vi "Apply ROIs.vi"(5 "Function":T1=enum."Write-from dataset", 7 "Mode (Redraw All)":enum16{"Redraw All", "Draw Last"}(ring), 8 "error in (no error)":errorcluster, 9 "ROIs Info []":T2[](array[typedef]) {"Zoom" min=1.0 max=10.0 step=0.10000000149011612}) -> (0 "error out":errorcluster, 1 "Number of ROI":i32, 2 "Cycle time (us)":dbl, 3 "No ROI":bool)   [LabVIEW 2017]
uses:
  Typedefs/ROI spec.ctl
  Typedefs/ROI ID Enum.ctl
  Typedefs/ROI management FG states.ctl
  Typedefs/ROI management Input cluster.ctl
  Global Variables/General Globals.vi
  <resource>/objmgr/IMAQImage.rc
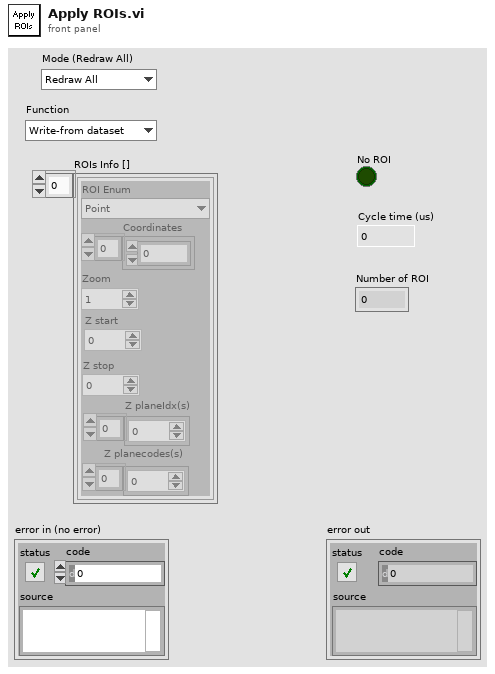
[diagram p1: front panel]
types:
  T1 = typedef "ROI management FG states.ctl" = enum16{"Read", "Write", "Write-from dataset", "Clear Last", "Clear All", "Update ROIs time", "Reload last ROI set", "Offset all ROI", "Offset visible ROI"}
  T2 = typedef "ROI spec.ctl" = cluster{"Coordinates":i32[], "Zoom":dbl, "ROI Enum":T3, "Z planeIdx(s)":i32[], "Z planecodes(s)":u8[], "Z start":dbl, "Z stop":dbl}
  T3 = typedef "ROI ID Enum.ctl" = enum16{"Point", "MiniScan", "Comp. MiniScan", "Rectangle", "Comp. volume", "Arb. plane point", "None"}
  T4 = typedef "ROI parameters data type.ctl" = cluster{"ROI index":dbl, "ROI ID":dbl, "ROI Time (ns)":dbl, "Pixels in ROI":dbl, "X start":dbl, "Y start":dbl, "Z start":dbl, "X stop":dbl, "Y stop":dbl, "Z stop":dbl, "Angle (deg)":dbl, "Composite ID":dbl, "Number of lines":dbl, "Frame Size":dbl, "Zoom":dbl, "Laser Power (%)":dbl, "ROI group ID":dbl, "Z Plane Idx":i32[], "Z Plane codes":i32[]}
  T5 = typedef "ROI management Input cluster.ctl" = cluster{"ROI Type":T3, "XY Coordinates":i32[], "Motor Z Planes":dbl[], "Dwell time per POI or per pixel (us)":dbl, "Frame size":i32, "Zoom":dbl, "Z Plane Idx(s)":i32[], "Z Plane codes":u8[], "Z start":dbl, "Z stop":dbl}
  T6 = typedef "IMAQ Image.ctl" = refnum<image>
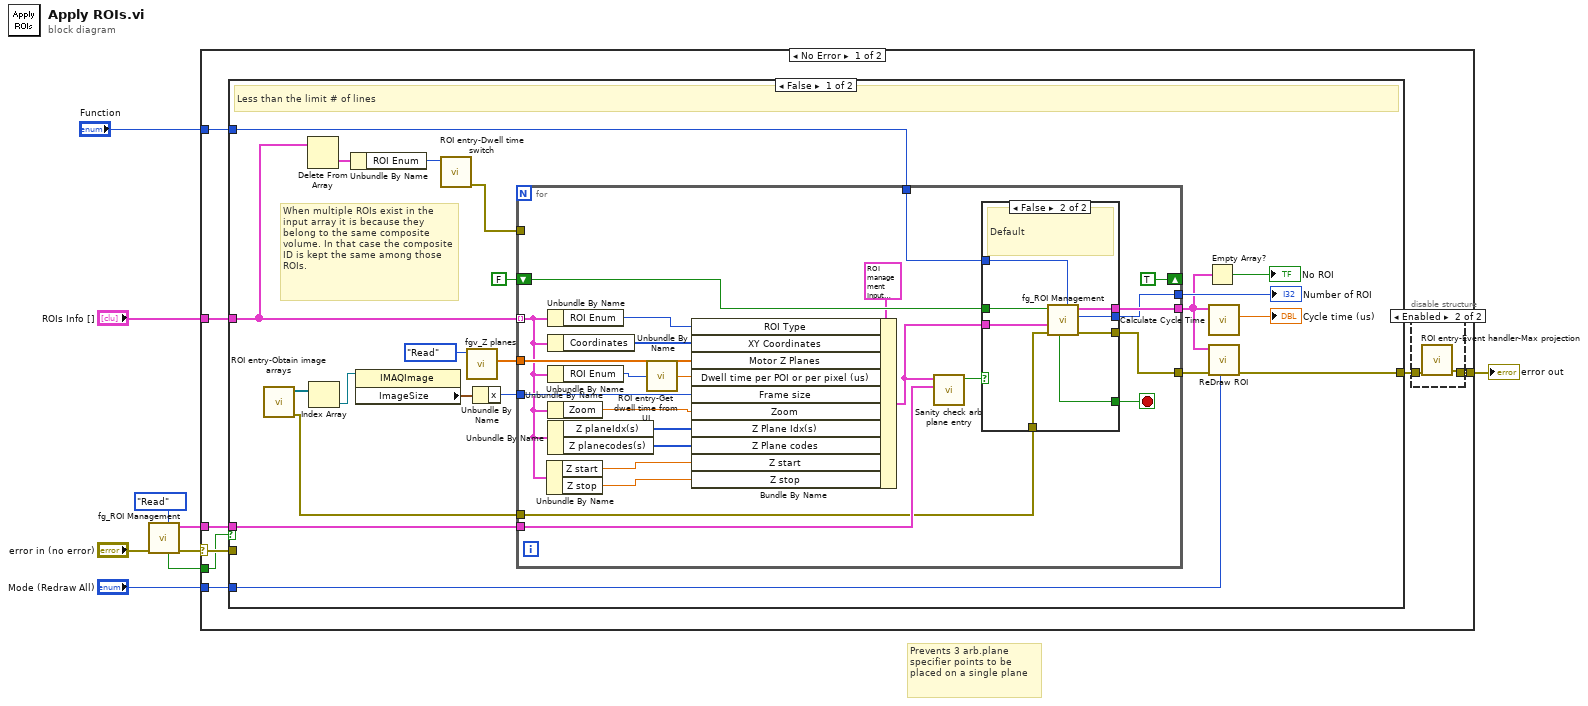
[diagram p0: block diagram]
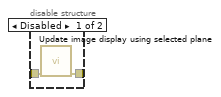
[diagram p2: hidden frame]
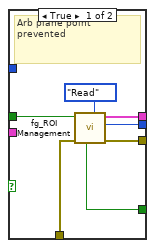
[diagram p3: hidden frame]
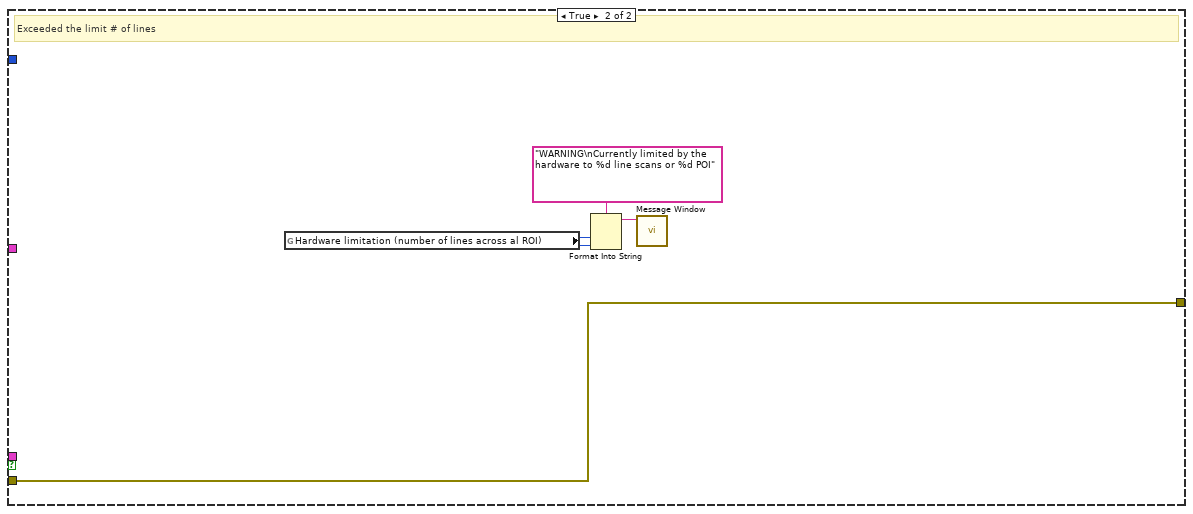
[diagram p4: hidden frame]
diagram:
  # "Prevents 3 arb.plane specifier points to be placed on a single plane"
  n1 = call "fg_ROI Management.vi"("Function"=ROI_management_FG_states."Read", "error in (no error)"="error in (no error)") -> ("error out"=w5:errorcluster, "ROI Setup"=w6:T4[], "No lines left"=w1:bool)  [unwired: 4 in, 3 out]
  n2 = case shown="No Error" w5 {
    selector: w5 -> [w15 w86]
    tunnel: w6 -> [w17 _]
    tunnel: [w13 w86] -> w4
    tunnel: "ROIs Info []" -> [w16 _]
    tunnel: "Mode (Redraw All)" -> [w12 _]
    tunnel: "Function" -> [w11 _]
    tunnel: w1 -> [w10 _]
    frame No Error {
      n3 = case shown="False" w10 {
        tunnel: w17 -> [w36 _]
        tunnel: w16 -> [w26 _]
        tunnel: [w32 w85] -> w14
        tunnel: w15 -> [_ w85]
        tunnel: w12 -> [w27 _]
        tunnel: w11 -> [w22 _]
        frame False {
          # "When multiple ROIs exist in the input array it is because they belong to the same composite volume. In that case the composite ID is kept the same among those ROIs."
          # "Less than the limit # of lines"
          n4 = call "ROI entry-Obtain image arrays.vi"() -> ("error IO"=w31:errorcluster, "RedImageArray"=w35:T6[])  [unwired: 10 in]
          n5 = Delete From Array(array=w26) -> (deleted portion=w25:T2)  [unwired: 2 in, 1 out]
          n6 = Index Array(array=w35) -> (element=w40:T6)  [unwired: 1 in]
          n7 = Unbundle By Name(w25) -> ("ROI Enum"=w24:T3)
          n8 = property class="IMAQImage"(reference=w40) -> ("ImageSize"=w39:cluster{"x":i32, "y":i32})  [unwired: 1 in, 2 out]
          n9 = call "ROI entry-Dwell time switch.vi"("ROI Enum"=w24) -> ("error out"=w23:errorcluster)  [unwired: 10 in]
          n10 = call "fgv_Z planes.vi"("Function"=enum16{"Intialize", "Write", "Read", "Clear"}."Read") -> ("AOL Z Planes"=w33:dbl[])  [unwired: 8 in, 2 out]
          n11 = Unbundle By Name(w39) -> ("x"=w38:i32)
          n12 = for {
            tunnel: [w66] -> w29
            tunnel: w26 -> [w46] mode=indexing
            tunnel: w33 -> [w62]
            shift-right: [TRUE] -> _
            shift-left: FALSE -> [w65]
            tunnel: w38 -> [w61]
            tunnel: [w57] -> w37
            tunnel: w36 -> [w55]
            tunnel: w31 -> [w53]
            tunnel: [w52] -> w30
            tunnel: w23 -> [_]
            tunnel: w22 -> [w43]
            stop <- w58 stop-if-true
            n13 = Unbundle By Name(w46) -> ("Z start"=w45:dbl, "Z stop"=w44:dbl)
            n14 = Unbundle By Name(w46) -> ("ROI Enum"=w51:T3)
            n15 = Unbundle By Name(w46) -> ("Coordinates"=w60:i32[])
            n16 = Unbundle By Name(w46) -> ("ROI Enum"=w49:T3)
            n17 = Unbundle By Name(w46) -> ("Zoom"=w59:dbl)
            n18 = Unbundle By Name(w46) -> ("Z planeIdx(s)"=w48:i32[], "Z planecodes(s)"=w47:u8[])
            n19 = call "ROI entry-Get dwell time from UI.vi"("ROI Enum"=w49) -> ("Dynamic dwell time(us)"=w50:dbl)
            n20 = Bundle By Name(cluster=T5 {"ROI Type"=enum."Point", "XY Coordinates"=[], "Motor Z Planes"=[], "Dwell time per POI or per pixel (us)"=0.0, "Frame size"=0, "Zoom"=0.0, "Z Plane Idx(s)"=[], "Z Plane codes"=[], "Z start"=0.0, "Z stop"=0.0} ("ROI management Input cluster"), "ROI Type"=w51, "XY Coordinates"=w60, "Motor Z Planes"=w62, "Dwell time per POI or per pixel (us)"=w50, "Frame size"=w61, "Zoom"=w59, "Z Plane Idx(s)"=w48, "Z Plane codes"=w47, "Z start"=w45, "Z stop"=w44) -> (w56:T5)
            n21 = call "Sanity check arb plane entry.vi"("ROI Setup"=w55, "ROI management Input cluster"=w56) -> ("Prevent new POI"=w54:bool)  [unwired: 9 in]
            n22 = case shown="False" w54 {
              tunnel: [w73 w81] -> w66
              tunnel: w65 -> [w72 w80]
              tunnel: [w71 w79] -> w58
              tunnel: [w69 w78] -> w57
              tunnel: w56 -> [_ w77]
              tunnel: w53 -> [w68 w76]
              tunnel: [w67 w75] -> w52
              tunnel: w43 -> [_ w74]
              frame True {
                # "Arb plane point prevented"
                n23 = call "fg_ROI Management.vi"("Function"=ROI_management_FG_states."Read", "error in (no error)"=w68, "Reuse last composite ID"=w72) -> ("error out"=w67:errorcluster, "Number of ROI"=w69:i32, "ROI Setup"=w73:T4[], "Exceeded limit number of lines"=w71:bool)  [unwired: 3 in, 2 out]
              }
              frame False {
                # "Default"
                n24 = call "fg_ROI Management.vi"("Function"=w74, "error in (no error)"=w76, "ROI management Input cluster"=w77, "Reuse last composite ID"=w80) -> ("error out"=w75:errorcluster, "Number of ROI"=w78:i32, "ROI Setup"=w81:T4[], "Exceeded limit number of lines"=w79:bool)  [unwired: 2 in, 2 out]
              }
            }
          }
          "Number of ROI" <- w37
          n25 = Empty Array?(array=w29) -> (empty?=→"No ROI":bool)
          n26 = call "Calculate Cycle Time.vi"("Coordinates"=w29) -> ("Cycle time (us)"=→"Cycle time (us)":dbl)  [unwired: 9 in, 1 out]
          n27 = call "ReDraw ROI.vi"("Mode (Redraw All)"=w27, "error in"=w30, "XYZ Coordinates"=w29) -> ("error out"=w32:errorcluster)  [unwired: 8 in]
        }
        frame True {
          # "Exceeded the limit # of lines"
          n28 = global read "General Globals.vi" "Hardware limitation (number of lines across al ROI)"() -> (w82:i32)
          n29 = Format Into String(format string="WARNING\nCurrently limited by the hardware to %d line scans or %d POI" ("Message string"), w82, w82) -> (resulting string=w83:string)  [unwired: 2 in, 1 out]
          n30 = call "Message Window.vi"("Message string"=w83) -> ()  [unwired: 10 in, 1 out]
        }
      }
      n31 = disable-structure shown="Enabled" {
        disable-tunnel: w14 -> [w19 w21]
        disable-tunnel: [w18 w20] -> w13
        frame Disabled {
          n32 = call "Update image display using selected plane.vi"("error in (no error)"=w19) -> ("error out"=w18:errorcluster)  [unwired: 10 in]
        }
        frame Enabled {
          n33 = call "ROI entry-Event handler-Max projection.vi"("error in (no error)"=w21) -> ("error out"=w20:errorcluster)  [unwired: 10 in]
        }
      }
    }
    frame Error {
    }
  }
  "error out" <- w4
